vi "Evaluate New Day.vi"(8 "error in (no error)":errorcluster, 11 "Text File Sink in":refnum<class "Text File Sink.lvclass">) -> (0 "error out":errorcluster, 3 "Text File Sink out":refnum<class "Text File Sink.lvclass">)   [LabVIEW 2016, in "Stream Log.lvlib" / "Text File Sink.lvclass"]
doc: "--\nCopyright © 2017 Composed SystemsI All rights reserved.\n\nAuthor: Jon McBee <jon.mcbee@composed.io>\n\nThis library is provided \"AS IS\" ,WITHOUT WARRANTIES OR\nCONDITIONS OF ANY KIND, either express or implied.\n\nComposed Systems -- composed.io\n\nStream 0.0.1.1\nJon McBee - Composed Systems\nCopyright (c) 2017, Composed Systems"
uses:
  <userlib>/Composed Systems/Stream/Log/Text File Sink/Text File Sink.lvclass
  <userlib>/Composed Systems/Stream/Log/Text File Sink/Text File Sink.lvclass/Text File Sink.ctl
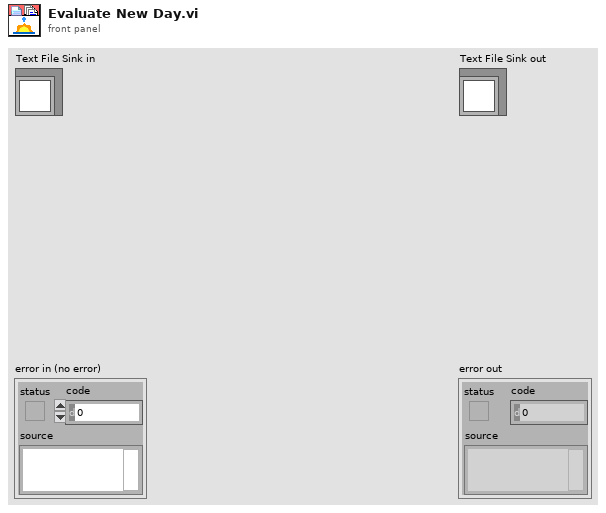
[diagram p1: front panel]
types:
  T1 = typedef "LVDateTimeRec.ctl" = cluster{"fractional second":dbl, "second":i32, "minute":i32, "hour":i32, "day of month":i32, "month":i32, "year":i32, "day of week":i32, "day of year":i32, "DST":i32}
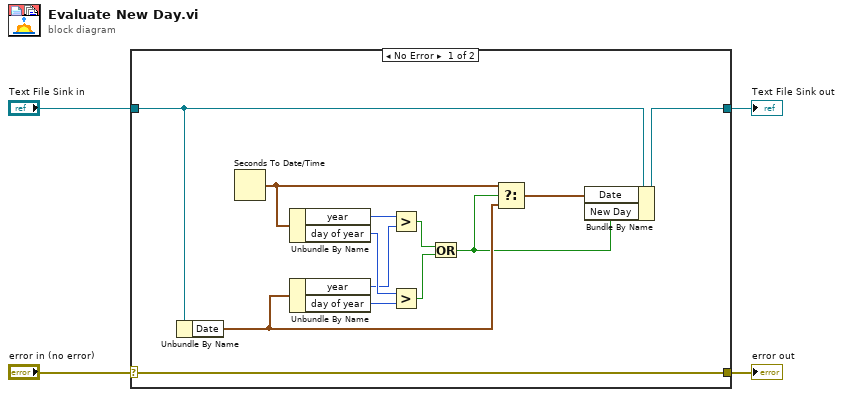
[diagram p0: block diagram]
diagram:
  n1 = case shown="No Error" "error in (no error)" {
    selector: "error in (no error)" -> [w17 w19]
    tunnel: [w17 w19] -> w3
    tunnel: [w5 w18] -> w1
    tunnel: "Text File Sink in" -> [w6 w18]
    frame No Error {
      n2 = Unbundle By Name(w6) -> ("Date"=w9:T1)
      n3 = Seconds To Date/Time() -> (date time rec=w16:T1)  [unwired: 2 out]
      n4 = Unbundle By Name(w16) -> ("year"=w15:i32, "day of year"=w14:i32)
      n5 = Unbundle By Name(w9) -> ("year"=w12:i32, "day of year"=w13:i32)
      n6 = Greater?(x=w15, y=w12) -> (0:w10:bool)
      n7 = Greater?(x=w14, y=w13) -> (0:w11:bool)
      n8 = Or(x=w10, y=w11) -> (x .or. y?=w7:bool)
      n9 = Select(t=w16, s=w7, f=w9) -> (s? t:f=w8:T1)
      n10 = Bundle By Name(cluster=w6, "Date"=w8, "New Day"=w7) -> (w5:refnum<class "Text File Sink.lvclass">)
    }
    frame Error {
    }
  }
  "error out" <- w3
  "Text File Sink out" <- w1
